vi "PRL BUFFER Rearrange Complex 2D Array.vi"(10 "Cut Index":i32, 11 "Array In":csg[][](array[numeric])) -> (3 "Array Out":csg[][](array[numeric]))   [LabVIEW 2018, in "S3DK.lvlib" / "PMU Recorder Light.lvlib"]
uses:
  PMU Recorder Light.lvlib
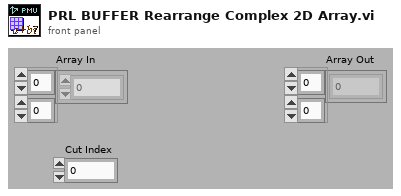
[diagram p1: front panel]
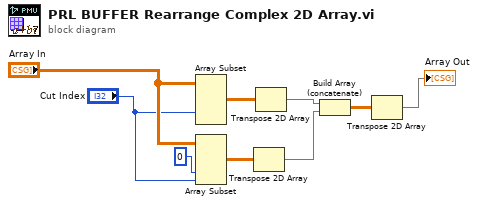
[diagram p0: block diagram]
diagram:
  n1 = Array Subset(array="Array In", index (col)="Cut Index") -> (w4:csg[][])  [unwired: 3 in]
  n2 = Array Subset(array="Array In", index (col)=0 ("index"), length (col)="Cut Index") -> (w9:csg[][])  [unwired: 2 in]
  n3 = Transpose 2D Array(2D array=w9) -> (transposed array=w2:csg[][])
  n4 = Transpose 2D Array(2D array=w4) -> (transposed array=w3:csg[][])
  n5 = Build Array (concatenate)(w3, w2) -> (w5:csg[][])
  n6 = Transpose 2D Array(2D array=w5) -> (transposed array=→"Array Out":csg[][])
